vi "get_attr_meta_dat.vi"(3 "NC_attrarray":T1(array[cluster])) -> (1 "NC_attr_meta_data_arr":cluster{"name":string, "xvalue":string}[](array[cluster]))   [LabVIEW 2016]
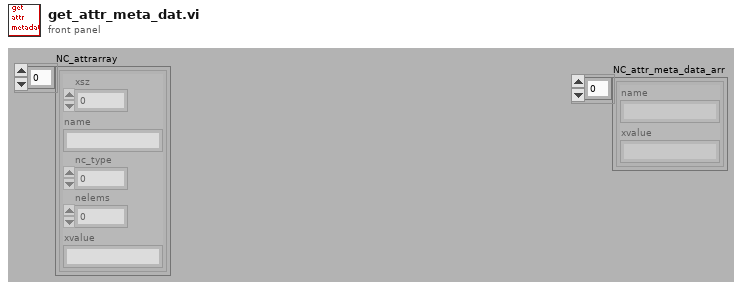
[diagram p1: front panel]
types:
  T1 = cluster{"xsz":u64, "name":string, "nc_type":u16, "nelems":u64, "xvalue":string}[]
  T2 = enum16{"big-endian, network order", "native, host order", "little-endian"}
  T3 = enum16{"NC_NAT", "NC_BYTE", "NC_CHAR", "NC_SHORT", "NC_INT", "NC_FLOAT", "NC_DOUBLE"}
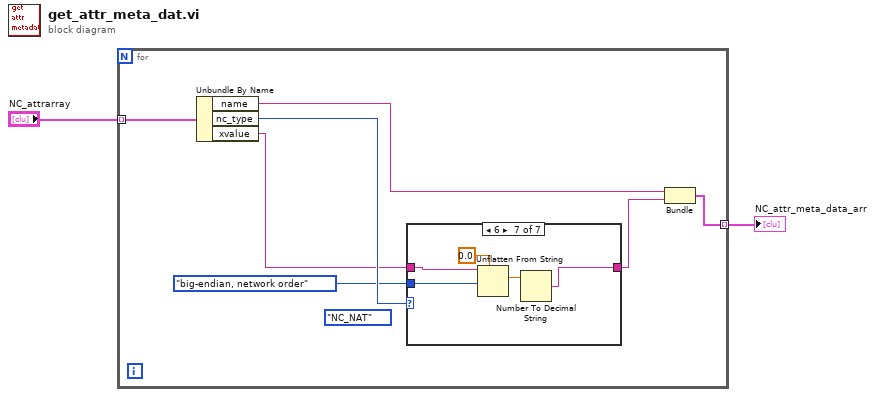
[diagram p0: block diagram]
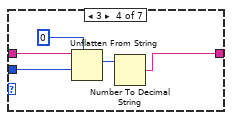
[diagram p5: hidden frame]
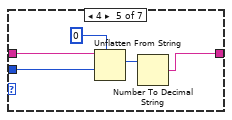
[diagram p6: hidden frame]
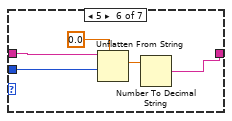
[diagram p7: hidden frame]
diagram:
  n1 = for {
    tunnel: "NC_attrarray" -> [w9] mode=indexing
    tunnel: [w4] -> w1 mode=indexing
    (unwired) T3."NC_NAT" ("nc_type")
    n2 = Unbundle By Name(w9) -> ("name"=w5:string, "nc_type"=w8:u16, "xvalue"=w7:string)
    n3 = case shown="6" w8 {
      tunnel: [w10 w11 w12 w15 w19 w24 w30] -> w3
      tunnel: w7 -> [w10 w11 w12 w16 w21 w26 w29]
      tunnel: T2."big-endian, network order" ("字节顺序(0:big-endian, network order)") -> [_ _ _ w13 w18 w23 w28]
      frame 0, Default {
      }
      frame 1 {
      }
      frame 2 {
      }
      frame 3 {
        n4 = Unflatten From String(type=i16 0, binary string=w16, byte order (0:big-endian, network order)=w13) -> (value=w14:i16)  [unwired: 2 in, 2 out]
        n5 = Number To Decimal String(number=w14) -> (decimal integer string=w15:string)  [unwired: 1 out]
      }
      frame 4 {
        n6 = Unflatten From String(type=0, binary string=w21, byte order (0:big-endian, network order)=w18) -> (value=w22:i32)  [unwired: 2 in, 2 out]
        n7 = Number To Decimal String(number=w22) -> (decimal integer string=w19:string)  [unwired: 1 out]
      }
      frame 5 {
        n8 = Unflatten From String(type=sgl 0.0, binary string=w26, byte order (0:big-endian, network order)=w23) -> (value=w27:sgl)  [unwired: 2 in, 2 out]
        n9 = Number To Decimal String(number=w27) -> (decimal integer string=w24:string)  [unwired: 1 out]
      }
      frame 6 {
        n10 = Unflatten From String(type=0.0, binary string=w29, byte order (0:big-endian, network order)=w28) -> (value=w32:dbl)  [unwired: 2 in, 2 out]
        n11 = Number To Decimal String(number=w32) -> (decimal integer string=w30:string)  [unwired: 1 out]
      }
    }
    n12 = Bundle("name"=w5, "xvalue"=w3) -> (w4:cluster{"name":string, "xvalue":string})  [unwired: 1 out]
  }
  "NC_attr_meta_data_arr" <- w1
